vi "StoreSignalByName.vi"(10 "Stored Signal":T1, 11 "Signal Array Input":T1[](array[typedef])) -> (3 "Signal Array Output":T1[](array[typedef]))   [LabVIEW 2009]
uses:
  Ctrl_Signal.ctl
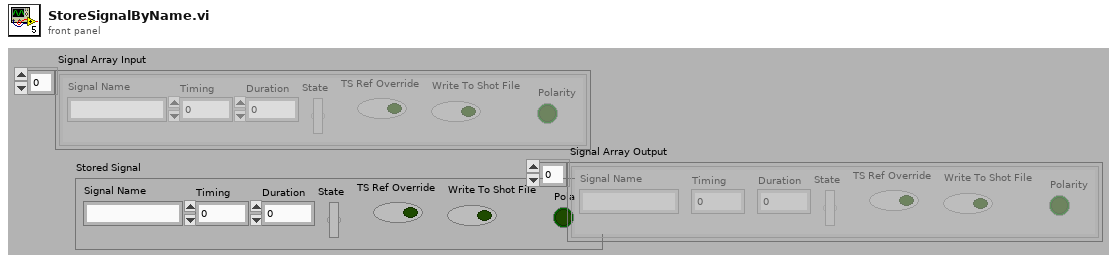
[diagram p1: front panel]
types:
  T1 = typedef "Ctrl_Signal.ctl" = cluster{"Signal Name":string, "Timing":dbl, "Duration":dbl, "State":bool, "TS Ref Override":bool, "Write To Shot File":bool, "Polarity":bool}
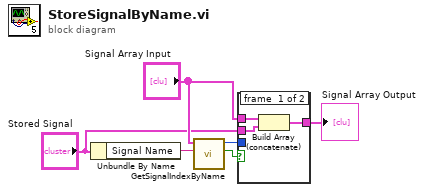
[diagram p0: block diagram]
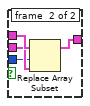
[diagram p2: hidden frame]
diagram:
  n1 = Unbundle By Name("Stored Signal") -> ("Signal Name"=w6:string)
  n2 = call "GetSignalIndexByName.vi"("Signal Name"=w6, "Signal Array In"="Signal Array Input") -> ("Signal Found"=w5:bool, "Index Out"=w1:u32)  [unwired: 8 in]
  n3 = case shown="False" w5 {
    tunnel: "Signal Array Input" -> [w9 w13]
    tunnel: [w7 w12] -> w3
    tunnel: "Stored Signal" -> [w8 w11]
    tunnel: w1 -> [_ w10]
    frame #0 {
      n4 = Build Array (concatenate)(w9, w8) -> (w7:T1[])
    }
    frame #1 {
      n5 = Replace Array Subset(array=w13, new element=w11, index=w10) -> (w12:T1[])
    }
  }
  "Signal Array Output" <- w3
